vi "Aggregate_Pupil_Data.vi"(8 "Subarray":sgl[](array[numeric]), 10 "Partial Sum R":dbl, 11 "Partial Sum  L":dbl) -> (2 "Sum R":dbl, 3 "Sum L":dbl)   [LabVIEW 2020]
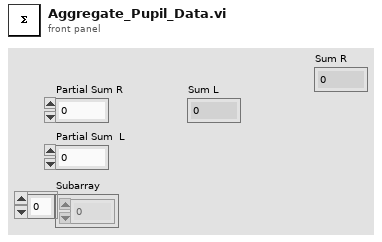
[diagram p1: front panel]
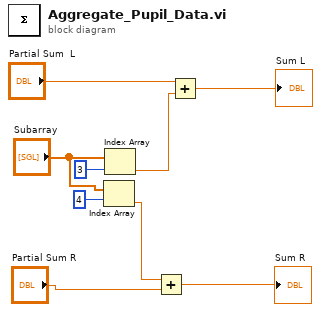
[diagram p0: block diagram]
diagram:
  n1 = Index Array(array="Subarray", index=4) -> (element=w2:sgl)
  n2 = Index Array(array="Subarray", index=3) -> (element=w5:sgl)
  n3 = Add(x=w2, y="Partial Sum R") -> (x+y=→"Sum R":dbl)
  n4 = Add(x="Partial Sum  L", y=w5) -> (x+y=→"Sum L":dbl)
